vi "prueba sonido.vi"() -> ()   [LabVIEW 2010]
uses:
  <vilib>/sound2/lvsound2.llb/Sound Data Format.ctl
  <vilib>/sound2/lvsound2.llb/Sampling Mode.ctl
  <vilib>/sound2/lvsound2.llb/Sound Output Write (DBL Single).vi
panel:
  out "XY Graph":cluster{sgl[], dbl[]}(graph)
  out "size(s)":i32
  in  "miu (ms)":u32
  in  "Sigma (ms)":u32
  in  "Amplitud":dbl
  out "1/x":sgl
  out "x*y":dbl
  out "#samples":u32
  in  "frequency":dbl=10.0 format="%0.2p"
  out "Generated Sound":waveform(dbl)(graph)={"t0"=timestamp(1.2471655328798186 s since 1904-01-01), "dt"=2.2675736961451248e-05, "Y"=[]}
  in  "sound format":T1={"sample rate (S/s)"=22050.0, "number of channels"=2, "bits per sample"=16}
  in  "tiempo (ms)":u32=100
  in  "stop 2":bool
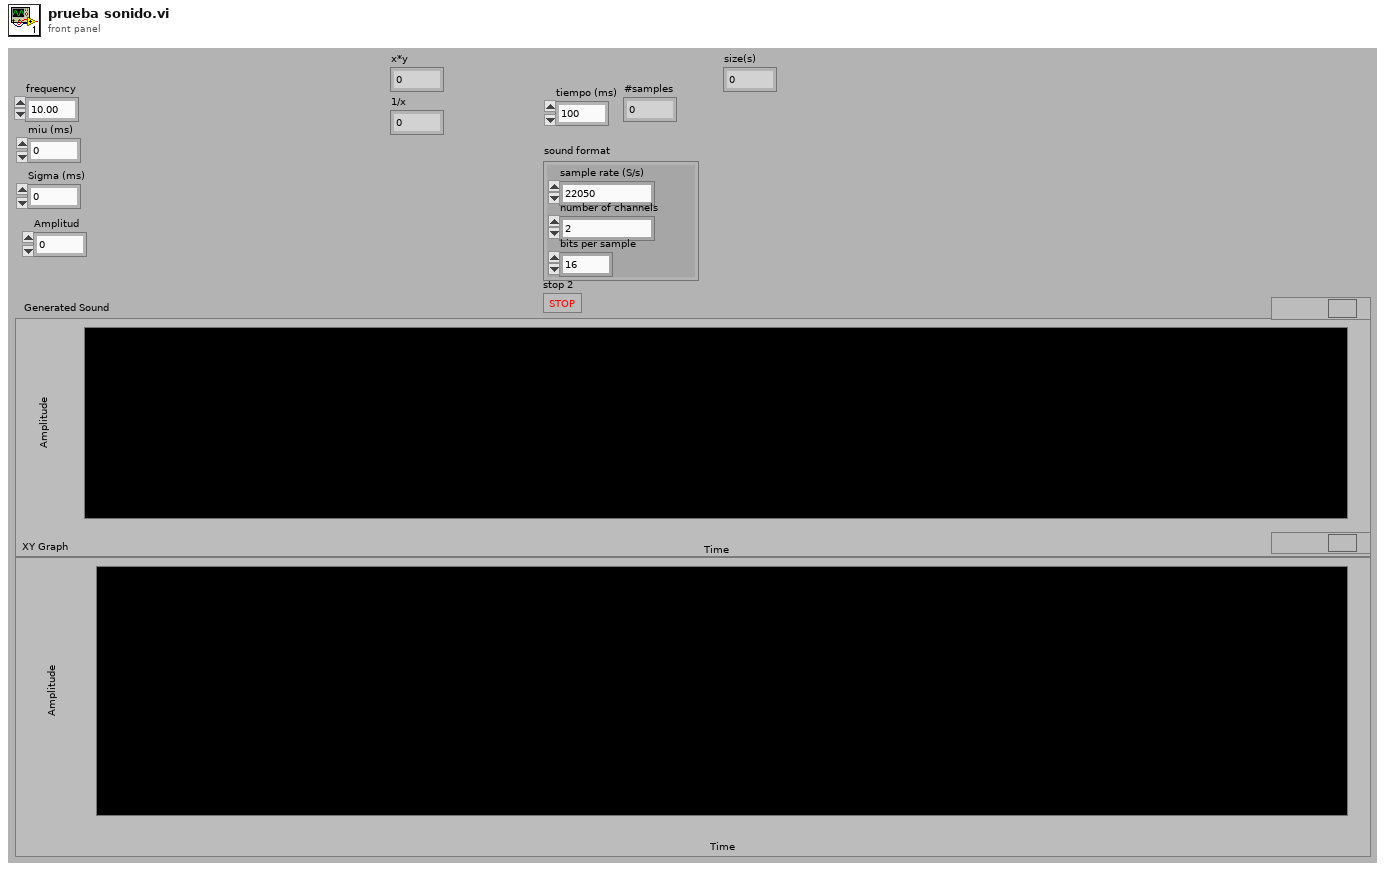
[diagram p1: front panel]
types:
  T1 = typedef "Sound Data Format.ctl" = cluster{"sample rate (S/s)":dbl, "number of channels":i32, "bits per sample":i32}
  T2 = typedef "Sampling Mode.ctl" = i32
  T3 = typedef "Sound Output Task ID.ctl" = u32
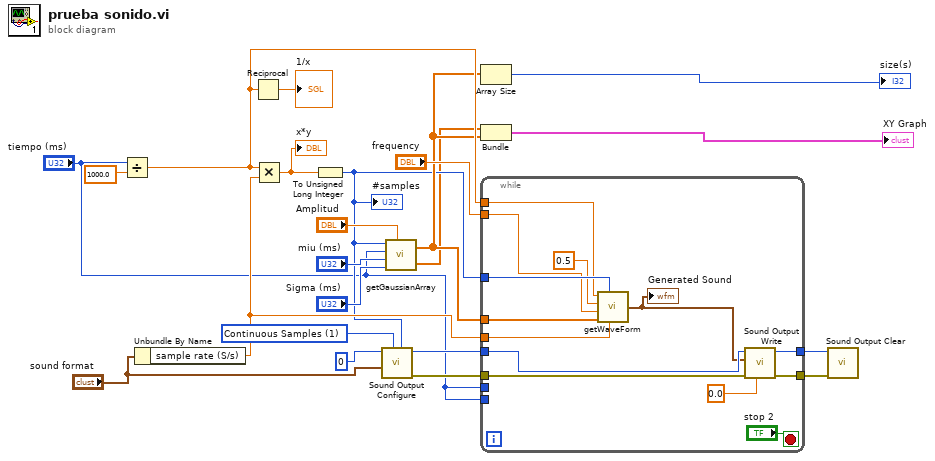
[diagram p0: block diagram]
diagram:
  w22 = T2 1 items=["Finite Samples", "Continuous Samples"] ("sample mode")
  n1 = Divide(x="tiempo (ms)", y=sgl 1000.0) -> (x/y=w9:sgl)
  n2 = Unbundle By Name("sound format") -> ("sample rate (S/s)"=w13:dbl)
  n3 = Reciprocal(x=w9) -> (1/x=→"1/x":sgl)
  n4 = Multiply(x=w9, y=w13) -> (x*y=w12:dbl)
  "x*y" <- w12
  n5 = To Unsigned Long Integer(number=w12) -> (unsigned 32bit integer=w4:u32)
  "#samples" <- w4
  n6 = call <vilib>:"Sound Output Configure.vi"("number of samples/ch"=w4, "sample mode"=w22, "sound format"="sound format", "device ID"=u32 0) -> ("error out"=w19:errorcluster, "task ID"=w20:T3)  [unwired: 6 in]
  n7 = call "getGaussianArray.vi"("#samples"=w4, "tiempo (ms)"="tiempo (ms)", "miu (ms)"="miu (ms)", "Sigma (ms)"="Sigma (ms)", "Amplitud"="Amplitud") -> ("Y out"=w5:dbl[], "t out"=w3:sgl[])
  n8 = Array Size(array=w5) -> (size(s)=→"size(s)":i32)
  n9 = Bundle("t out"=w3, "Y out"=w5) -> (→"XY Graph":cluster{"t out":sgl[], "Y out":dbl[]})  [unwired: 1 in]
  n10 = while {
    tunnel: w20 -> [w35]
    tunnel: w19 -> [w34]
    tunnel: [w33] -> w18
    tunnel: [w32] -> w17
    tunnel: "tiempo (ms)" -> [_]
    tunnel: "frequency" -> [w25]
    tunnel: w13 -> [w29]
    tunnel: w4 -> [w28]
    tunnel: w9 -> [w26]
    tunnel: "tiempo (ms)" -> [_]
    tunnel: w5 -> [w23]
    stop <- "stop 2" stop-if-true
    n11 = call "getWaveForm.vi"("tiempo (s)"=w26, "#samples"=w28, "Amplitud"=0.5, "frecuencia"=w25, "Fs (S/s)"=w29, "df"=w23) -> ("Waveform"=w30:waveform(dbl))  [unwired: 2 out]
    "Generated Sound" <- w30
    n12 = call-poly <vilib>:"Sound Output Write.vi"("timeout (sec)"=0.0, "error in (no error)"=w34, "data"=w30, "task ID"=w35) -> ("error out"=w32:errorcluster, "task ID out"=w33:T3)  [unwired: 6 in]
  }
  n13 = call <vilib>:"Sound Output Clear.vi"("error in (no error)"=w17, "task ID"=w18) -> ()  [unwired: 9 in, 1 out]
